vi "MultiChannelType_Image.vi"(9 "error in":errorcluster, 11 "Image Reference":T2) -> (1 "error out":errorcluster, 2 "MultiChannelType":T1, 3 "Image Reference":T2)   [LabVIEW 2020, in "OpenLvVision_OpenCv.lvlib"]
uses:
  OpenLvVision_OpenCv.lvlib
  <vilib>/OpenLvVision/OpenLvVision_Image/Management/TypeDef/OLV Image.ctl
  <vilib>/OpenLvVision/OpenLvVision_Image/Management/TypeDef/OLV ImageType.ctl
  <vilib>/Utility/error.llb/Error Cluster From Error Code.vi
  <vilib>/ErrorRing/Error Ring.xnode
  <vilib>/OpenLvVision/OpenLvVision_Image/Management/OLV Management.lvlib
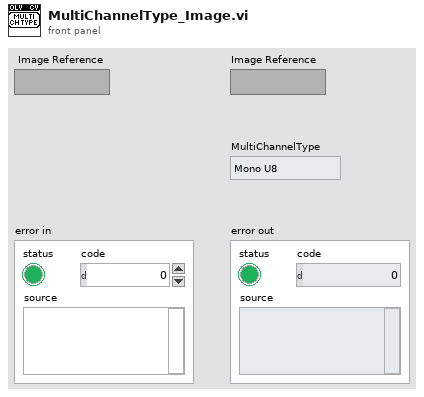
[diagram p1: front panel]
types:
  T1 = typedef "OLV OpenLvVision_Image.lvlib/OLV Management.lvlib/OLV ImageType.ctl" = enum16{"Mono U8", "Mono U16", "Mono I16", "Mono SGL", "Color U32", "Color U64", "Complex CSG"}
  T2 = typedef "OLV OpenLvVision_Image.lvlib/OLV Management.lvlib/OLV Image.ctl" = refnum<image>
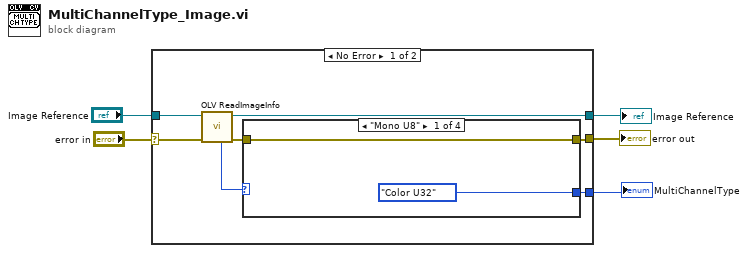
[diagram p0: block diagram]
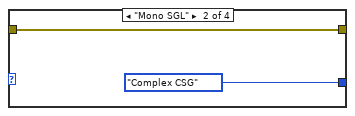
[diagram p2: hidden frame]
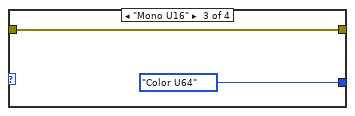
[diagram p3: hidden frame]
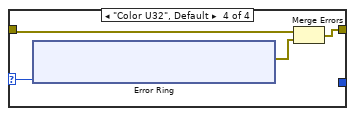
[diagram p4: hidden frame]
diagram:
  n1 = case shown="No Error" "error in" {
    selector: "error in" -> [w11 w30]
    tunnel: "Image Reference" -> [w12 w31]
    tunnel: [w10 w31] -> w2
    tunnel: [w6 w30] -> w4
    tunnel: [w8 _] -> w1
    frame No Error {
      n2 = call <vilib>:"OLV ReadImageInfo.vi"("error in"=w11, "Image Reference In"=w12) -> ("error out"=w7:errorcluster, "Image Reference Out"=w10:T2, "Image Type"=w9:T1)  [unwired: 4 in, 3 out]
      n3 = case shown="\"Mono U8\"" w9 {
        selector: w9 -> [_ _ _ w22]
        tunnel: [OLV_ImageType."Color U32" ("Image Type") OLV_ImageType."Complex CSG" ("Image Type") OLV_ImageType."Color U64" ("Image Type") _] -> w8
        tunnel: w7 -> [w13 w16 w17 w21]
        tunnel: [w13 w16 w17 w19] -> w6
        frame "Mono U8" {
        }
        frame "Mono SGL" {
        }
        frame "Mono U16" {
        }
        frame "Color U32", Default {
          n4 = xnode "Error Ring"("parameter 0"=w22) -> ("error out"=w20:errorcluster)
          n5 = Merge Errors(w21, w20) -> (w19:errorcluster)
        }
      }
    }
    frame Error {
    }
  }
  "error out" <- w4
  "Image Reference" <- w2
  "MultiChannelType" <- w1
